vi "UWGN ident.vi"() -> ()   [LabVIEW 2015]
uses:
  <vilib>/FPGAPlugInAG/myRIO-1900/niLvFpga_Open_myRIO-1900.vi
  <vilib>/rvi/interface/common/dynamic/niFpgaDynamicAddResources.vi
  <vilib>/Utility/file.llb/Write Delimited Spreadsheet (DBL).vi
  <vilib>/Utility/error.llb/Error Cluster From Error Code.vi
  <vilib>/rvi/errors/niLvFpgaAdjustHostInterfaceError.vi
  <vilib>/FPGAPlugInAG/Dynamic/niLvFpga_Close_Dynamic.vi
  <vilib>/rvi/interface/nirviOpenFPGA/nirviOpenFPGA.xnode
  FPGA Bitfiles/ACC20115_FPGATarget_CurrentControlle_Dt5vFgOzYtY.lvbitx
  Current Controller.vi
  <vilib>/rvi/interface/nirviReadWriteControl/nirviReadWriteControl.xnode
  <vilib>/rvi/interface/nirviCloseFPGA/nirviCloseFPGA.xnode
  NiFpgaLv.dll
  <vilib>/rvi/interface/Simulation/niFpgaSimulationCallBeginRW.vi
  <vilib>/Analysis/NI_AALBase.lvlib
panel:
  out "error out":errorcluster
  in  "Stop":bool
  in  "Tab Control":enum32{"Monitor"}(tab)
  out "GU Wave":dbl[](graph)
  out "Sensor":dbl(graph)
  out "FPGA Status":bool
  out "ms":u32
  out "Sampling Frequency":dbl(graph)
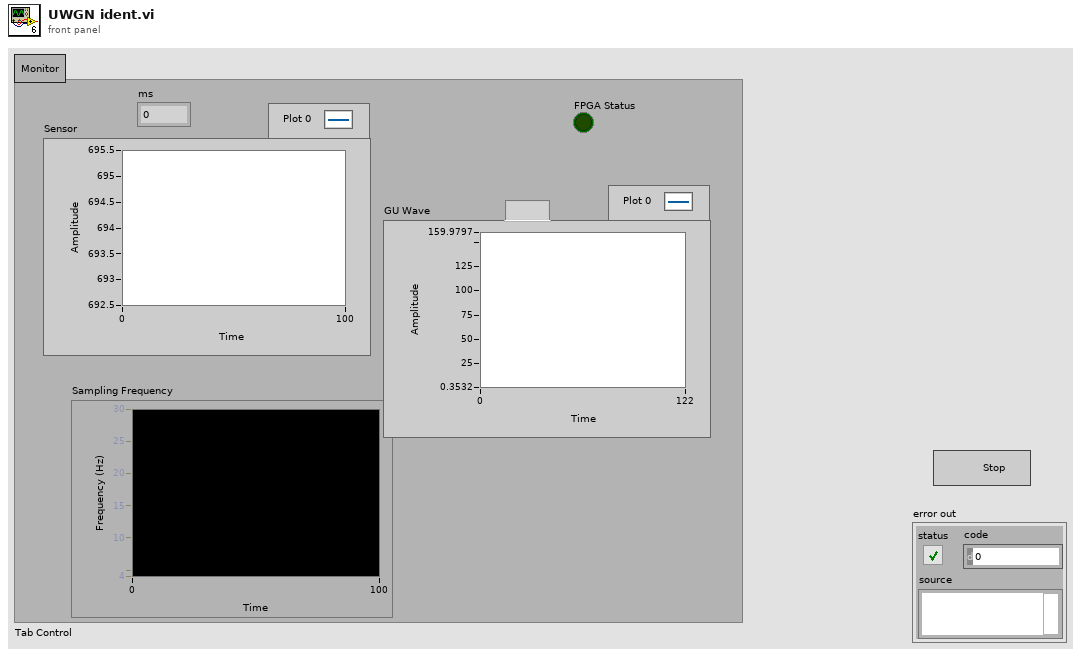
[diagram p1: front panel]
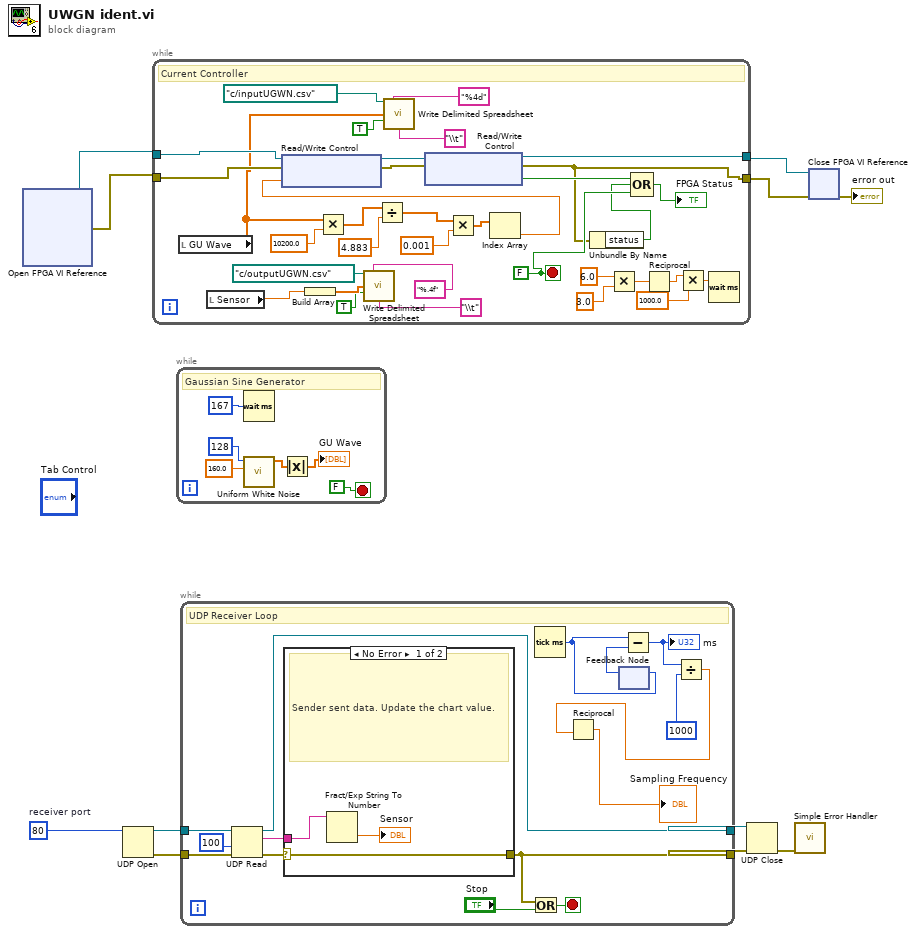
[diagram p0: block diagram]
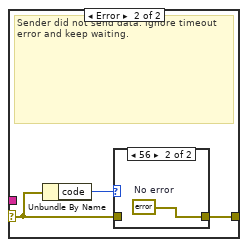
[diagram p2: hidden frame]
diagram:
  w2 = u16 80  # receiver port
  n1 = xnode "Open FPGA VI Reference"() -> ("FPGA VI Reference Out"=w11:refnum<k20>, "error out"=w10:errorcluster)  [unwired: 2 in]
  n2 = UDP Open(11:w2) -> (port=w3:refnum<k16>, 0:w4:errorcluster)  [unwired: 4 in, 1 out]
  n3 = while {
    tunnel: w11 -> [w45]
    tunnel: w10 -> [w44]
    tunnel: [w36] -> w9
    tunnel: [w32] -> w8
    stop <- w35 stop-if-true
    w35 = FALSE
    # "Current Controller"
    n4 = local read "GU Wave"() -> (w12:dbl[])
    n5 = local read "Sensor"() -> (w25:dbl)
    n6 = Build Array(w25) -> (w26:dbl[])
    n7 = Multiply(x=w12, y=10200.0) -> (x*y=w40:dbl[])
    n8 = call-poly <vilib>:"Write Delimited Spreadsheet.vi"("file path (dialog if empty)"=path "c:/outputUGWN.csv", "format (%.3f)"="%.4f", "1D data"=w26, "append to file? (F)"=TRUE, "delimiter (\\t)"="\\t" ("delimiter (\\t)")) -> ()  [unwired: 9 in, 2 out]
    n9 = Divide(x=w40, y=4.883) -> (x/y=w42:dbl[])
    n10 = call-poly <vilib>:"Write Delimited Spreadsheet.vi"("file path (dialog if empty)"=path "c:/inputUGWN.csv", "format (%.3f)"="%4d" ("format (%d)"), "1D data"=w12, "append to file? (F)"=TRUE, "delimiter (\\t)"="\\t" ("delimiter (\\t)")) -> ()  [unwired: 9 in, 2 out]
    n11 = Multiply(x=w42, y=0.001) -> (x*y=w20:dbl[])
    n12 = Index Array(array=w20) -> (element=w13:dbl)  [unwired: 1 in]
    n13 = xnode "Read/Write Control"("FPGA VI Reference In"=w45, "error in"=w44, "DAC Inlet Valve"=w13) -> ("FPGA VI Reference Out"=w38:refnum<k20>, "error out"=w37:errorcluster)
    n14 = xnode "Read/Write Control"("FPGA VI Reference In"=w38, "error in"=w37) -> ("FPGA VI Reference Out"=w36:refnum<k20>, "error out"=w32:errorcluster, "Inlet Overflow?"=w33:bool)
    n15 = Unbundle By Name(w32) -> ("status"=w34:bool)
    n16 = Multiply(x=6.0, y=3.0) -> (x*y=w17:dbl)
    n17 = Compound Arithmetic op=OR(w33, w34, w35) -> (→"FPGA Status":bool)
    n18 = Reciprocal(x=w17) -> (1/x=w15:dbl)
    n19 = Multiply(x=w15, y=1000.0) -> (x*y=w16:dbl)
    n20 = Wait (ms)(milliseconds to wait=w16) -> ()  [unwired: 1 out]
  }
  n21 = while {
    stop <- FALSE stop-if-true
    # "Gaussian Sine Generator"
    n22 = Wait (ms)(milliseconds to wait=u32 167) -> ()  [unwired: 1 out]
    n23 = call <vilib>:"Uniform White Noise.vi"("amplitude"=160.0, "samples"=128) -> ("uniform white noise"=w47:dbl[])  [unwired: 8 in, 1 out]
    n24 = Absolute Value(x=w47) -> (abs(x)=→"GU Wave":dbl[])
  }
  n25 = while {
    tunnel: w3 -> [w66]
    tunnel: [w58] -> w7
    tunnel: w4 -> [w63]
    tunnel: [w59] -> w5
    stop <- w64 stop-if-true
    # "UDP Receiver Loop"
    n26 = UDP Read(connection ID=w66, timeout ms (25000)=100, 8:w63) -> (data out=w61:string, error out=w60:errorcluster, 3:w58:refnum<k16>)  [unwired: 3 out]
    n27 = case shown="No Error" w60 {
      selector: w60 -> [w67 w71]
      tunnel: w61 -> [w69 _]
      tunnel: [w67 w70] -> w59
      frame No Error {
        # "Sender sent data. Update the chart value."
        n28 = Fract/Exp String To Number(string=w69) -> (number=→"Sensor":dbl)  [unwired: 3 in, 1 out]
      }
      frame Error {
        # "Sender did not send data. Ignore timeout error and keep waiting."
        n29 = Unbundle By Name(w71) -> ("code"=w72:i32)
        n30 = case shown="56" w72 {
          tunnel: w71 -> [w73 _]
          tunnel: [w73 w74] -> w70
          frame Default {
          }
          frame 56 {
            w74 = errorcluster {"status"=FALSE, "code"=0, "source"=""}  # No error
          }
        }
      }
    }
    n31 = Or(x=w59, y="Stop") -> (x .or. y?=w64:bool)
    n32 = Tick Count (ms)() -> (millisecond timer value=w57:u32)
    n33 = feedback-in #1(w57) -> ()
    n34 = feedback #1() -> (w56:u32)  [unwired: 1 in]
    n35 = Subtract(x=w57, y=w56) -> (x-y=w54:u32)
    "ms" <- w54
    n36 = Divide(x=w54, y=u32 1000) -> (x/y=w53:dbl)
    n37 = Reciprocal(x=w53) -> (1/x=→"Sampling Frequency":dbl)
  }
  n38 = UDP Close(connection ID=w7, 8:w5) -> (error out=w6:errorcluster)  [unwired: 1 out]
  n39 = call <vilib>:"Simple Error Handler.vi"("error in (no error)"=w6) -> ()  [unwired: 1 in, 8 out]
  n40 = xnode "Close FPGA VI Reference"("FPGA VI Reference In"=w9, "error in"=w8) -> ("error out"=→"error out":errorcluster)
